vi "Injection Command Plot - TMP.vi"(10 "Injection Command":T1={"Mode"=enum."Off", "Digital Input"=enum."Unused", "Default Profile Index"=0, "Cal Freq [Hz]"=0.0, "Cal Duration [s]"=0.0, "Cal Increment [s]"=0.0, "Cal Pulses"=0, "TMP Command Sequence"=[{"Duration [s]"=0.0, "Level"=FALSE, "Run/Stop"=FALSE, "Profile Index"=0}, {"Duration [s]"=0.0, "Level"=FALSE, "Run/Stop"=FALSE, "Profile Index"=0}, {"Duration [s]"=0.0, "Level"=FALSE, "Run/Stop"=FALSE, "Profile Index"=0}, {"Duration [s]"=0.0, "Level"=FALSE, "Run/Stop"=FALSE, "Profile Index"=0}, {"Duration [s]"=0.0, "Level"=FALSE, "Run/Stop"=FALSE, "Profile Index"=0}, {"Duration [s]"=0.0, "Level"=FALSE, "Run/Stop"=FALSE, "Profile Index"=0}, {"Duration [s]"=0.0, "Level"=FALSE, "Run/Stop"=FALSE, "Profile Index"=0}, {"Duration [s]"=0.0, "Level"=FALSE, "Run/Stop"=FALSE, "Profile Index"=0}], "EPT TDC Offset [CAD]"=0.0, "EPT Window Start [DBTDC]"=0.0, "EPT Window End [DBTDC]"=0.0, "EPT Angles"=[{"Enable"=FALSE, "Timing [DBTDC]"=0.0, "Duration [s]"=0.0, "Profile Index"=0}, {"Enable"=FALSE, "Timing [DBTDC]"=0.0, "Duration [s]"=0.0, "Profile Index"=0}, {"Enable"=FALSE, "Timing [DBTDC]"=0.0, "Duration [s]"=0.0, "Profile Index"=0}, {"Enable"=FALSE, "Timing [DBTDC]"=0.0, "Duration [s]"=0.0, "Profile Index"=0}, {"Enable"=FALSE, "Timing [DBTDC]"=0.0, "Duration [s]"=0.0, "Profile Index"=0}, {"Enable"=FALSE, "Timing [DBTDC]"=0.0, "Duration [s]"=0.0, "Profile Index"=0}, {"Enable"=FALSE, "Timing [DBTDC]"=0.0, "Duration [s]"=0.0, "Profile Index"=0}, {"Enable"=FALSE, "Timing [DBTDC]"=0.0, "Duration [s]"=0.0, "Profile Index"=0}], "EPT Skip Fire"=FALSE, "EPT Skip Index"=0, "EPT Precharge Duration [s]"=0.0, "EPT Precharge Profile Index"=0} {"EPT Precharge Profile Index" max=15; "EPT Precharge Duration [s]" min=0 format="%#_4p"; "Default Profile Index" max=15; "Cal Increment [s]" format="%#_3p"; "TMP Command Sequence"."Profile Index" max=7; "TMP Command Sequence"."Duration [s]" min=0 max=100 format="%#_3p"; "Cal Pulses" max=511; "EPT Skip Index" max=7; "EPT Angles"."Profile Index" max=7; "EPT Angles"."Duration [s]" min=0 max=100 format="%#_3p"; "Cal Duration [s]" format="%#_3p"; "Cal Freq [Hz]" format="%#_3p"}) -> (2 "Plot":cluster{"Array":sgl[], "Array":sgl[]}[](array[cluster]))   [LabVIEW 2016]
uses:
  <vilib>/Powertrain Controls/Device Drivers/DCM/DI/RT/Command.ctl
  <vilib>/Powertrain Controls/Device Drivers/DCM/DI/FPGA/Mode.ctl
  <vilib>/Powertrain Controls/Device Drivers/DCM/Rev0/FPGA/Digital Channel.ctl
  <vilib>/Powertrain Controls/Device Drivers/DCM/DI/RT/Command Sequence.ctl
  <vilib>/Powertrain Controls/Device Drivers/DCM/DI/RT/Angle Control.ctl
  <vilib>/Powertrain Controls/Device Drivers/DCM/DI/FPGA/DCM - FPGA - DI.lvlib
  <vilib>/Powertrain Controls/Device Drivers/DCM/Rev0/FPGA/DCM - FPGA.lvlib
  <vilib>/Powertrain Controls/Device Drivers/DCM/DI/RT/DCM - RT - DI.lvlib
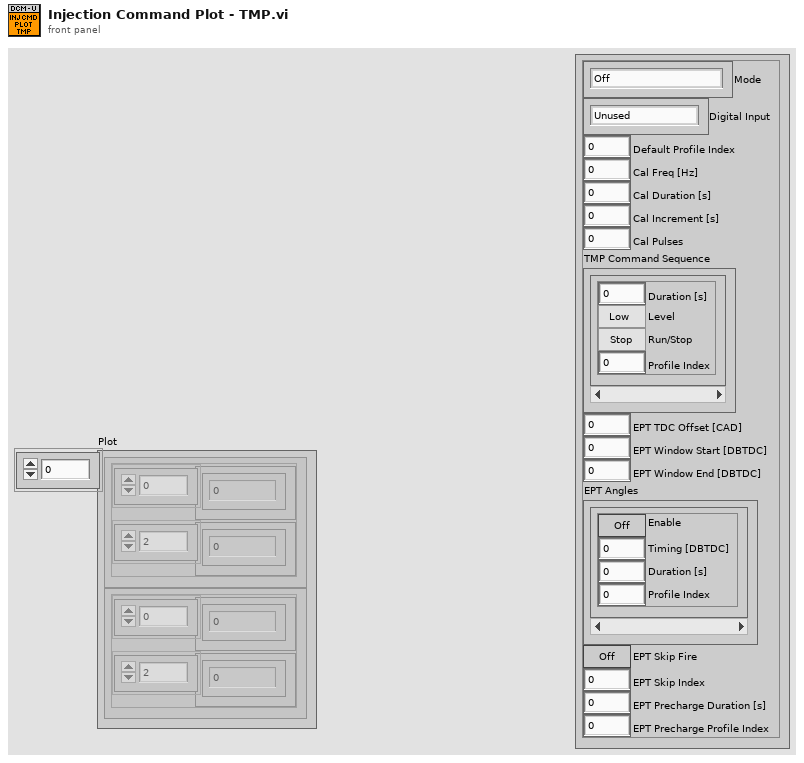
[diagram p1: front panel]
types:
  T1 = typedef "DCM - RT - DI.lvlib/Command.ctl" = cluster{"Mode":T2, "Digital Input":T3, "Default Profile Index":u8, "Cal Freq [Hz]":sgl, "Cal Duration [s]":sgl, "Cal Increment [s]":sgl, "Cal Pulses":u16, "TMP Command Sequence":T4[], "EPT TDC Offset [CAD]":sgl, "EPT Window Start [DBTDC]":sgl, "EPT Window End [DBTDC]":sgl, "EPT Angles":T5[], "EPT Skip Fire":bool, "EPT Skip Index":u8, "EPT Precharge Duration [s]":sgl, "EPT Precharge Profile Index":u8}
  T2 = typedef "DCM - FPGA - DI.lvlib/Mode.ctl" = enum8{"Off", "Direct", "Calibration", "Triggered Multi-Pulse", "Engine Position Tracking"}
  T3 = typedef "DCM - FPGA.lvlib/Digital Channel.ctl" = enum8{"Unused", "User OS", "Diff IO 1", "Diff IO 2", "Diff IO 3", "Diff IO 4", "Diff IO 5", "Diff IO 6", "Diff IO 7", "Diff IO 8", "Aux 1", "Aux 2", "Aux 3", "Aux 4", "Aux 5", "Aux 6", "Aux 7", "Aux 8", "Aux 9", "Aux 10", "Aux 11", "Aux 12", "Aux 13", "Aux 14", "Aux 15", "Aux 16"}
  T4 = typedef "DCM - RT - DI.lvlib/Command Sequence.ctl" = cluster{"Duration [s]":sgl, "Level":bool, "Run/Stop":bool, "Profile Index":u8}
  T5 = typedef "DCM - RT - DI.lvlib/Angle Control.ctl" = cluster{"Enable":bool, "Timing [DBTDC]":sgl, "Duration [s]":sgl, "Profile Index":u8}
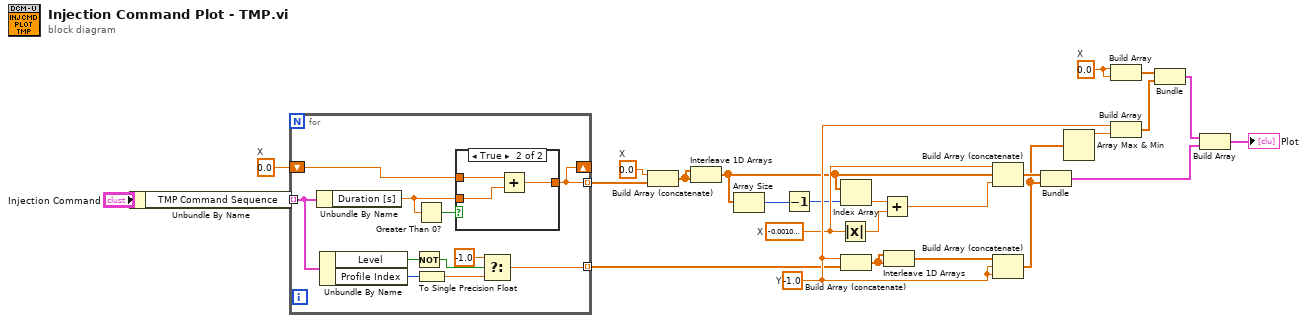
[diagram p0: block diagram]
diagram:
  w1 = sgl 0.0  # X
  w2 = sgl 0.0  # X
  w10 = sgl 0.0  # X
  w23 = sgl -1.0  # Y
  w22 = sgl -0.001  # X
  n1 = Unbundle By Name("Injection Command") -> ("TMP Command Sequence"=w4:T4[])
  n2 = for {
    tunnel: w4 -> [w35] mode=indexing
    shift-right: [w28] -> _
    shift-left: w1 -> [w29]
    tunnel: [w28] -> w5 mode=indexing
    tunnel: [w30] -> w6 mode=indexing
    n3 = Unbundle By Name(w35) -> ("Duration [s]"=w36:sgl)
    n4 = Unbundle By Name(w35) -> ("Level"=w33:bool, "Profile Index"=w34:u8)
    n5 = Not(x=w33) -> (.not. x?=w27:bool)
    n6 = Greater Than 0?(x=w36) -> (x > 0?=w37:bool)
    n7 = To Single Precision Float(number=w34) -> (single precision float=w32:sgl)
    n8 = case shown="True" w37 {
      tunnel: w36 -> [_ w41]
      tunnel: w29 -> [w38 w40]
      tunnel: [w38 w39] -> w28
      frame False {
      }
      frame True {
        n9 = Add(x=w40, y=w41) -> (x+y=w39:sgl)
      }
    }
    n10 = Select(t=sgl -1.0 ("Y"), s=w27, f=w32) -> (s? t:f=w30:sgl)
  }
  n11 = Build Array (concatenate)(w10, w5) -> (w9:sgl[])
  n12 = Interleave 1D Arrays(w9, w9) -> (w15:sgl[])
  n13 = Array Size(array=w15) -> (size(s)=w12:i32)
  n14 = Decrement(x=w12) -> (x-1=w13:i32)
  n15 = Absolute Value(x=w22) -> (abs(x)=w16:sgl)
  n16 = Index Array(array=w15, index=w13) -> (element=w14:sgl)
  n17 = Build Array (concatenate)(w23, w6) -> (w7:sgl[])
  n18 = Add(x=w14, y=w16) -> (x+y=w17:sgl)
  n19 = Interleave 1D Arrays(w7, w7) -> (w11:sgl[])
  n20 = Build Array (concatenate)(w22, w15, w17) -> (w8:sgl[])
  n21 = Build Array (concatenate)(w11, w23, w23) -> (w3:sgl[])
  n22 = Bundle(w8, w3) -> (w18:cluster{sgl[], sgl[]})  [unwired: 1 in]
  n23 = Array Max & Min(array=w3) -> (max value=w24:sgl)  [unwired: 3 out]
  n24 = Build Array(w2, w2) -> (w19:sgl[])
  n25 = Build Array(w23, w24) -> (w20:sgl[])
  n26 = Bundle(w19, w20) -> (w21:cluster{sgl[], sgl[]})  [unwired: 1 in]
  n27 = Build Array(w21, w18) -> (→"Plot":cluster{sgl[], sgl[]}[])
